vi "VarArray_Find elements.vi"(8 "Error In":errorcluster, 9 "Select Array In":variant[](array[variant]), 11 "Array In":variant[](array[variant])) -> (0 "Error Out":errorcluster, 1 "Selected Array Out":variant[](array[variant]), 2 "Index Array Out":i32[](array[numeric]), 3 "Array Out":variant[](array[variant]))   [LabVIEW 2015]
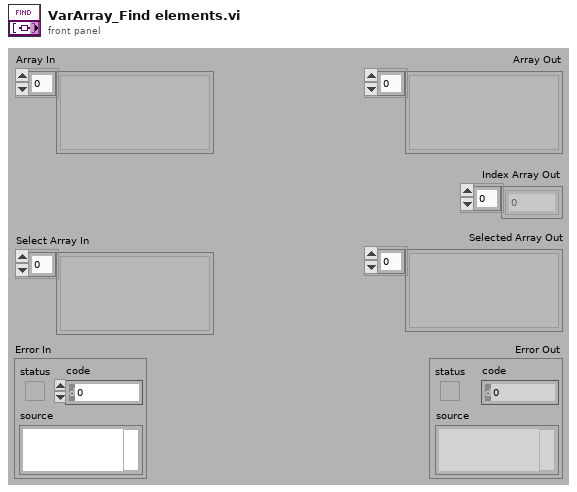
[diagram p1: front panel]
types:
  T1 = typedef "Type Descriptor Enumeration.ctl" = enum8{"<Null>", "I8", "I16", "I32", "I64", "U8", "U16", "U32", "U64", "SGL", "DBL", "EXT", "CSG", "CDB", "CXT", "0x0F", "0x10", "0x11", "0x12", "0x13", "0x14", "Enum U8", "Enum U16", "Enum U32", "Enum U64", "SGL PQ", "DBL PQ", "EXT PQ", "CSG PQ", "CDB PQ", "CXT PQ", "0x1F", "0x20", "Boolean", "0x22", "0x23", "0x24", "0x25", "0x26", "0x27", "0x28", "0x29", "0x2A", "0x2B", "0x2C", "0x2D", "0x2E", "0x2F", "String", "0x31", "Path", "Pict", "0x34", "0x35", "0x36", "DAQ", "0x38", "0x39", "0x3A", "0x3B", "0x3C", "0x3D", "0x3E", "0x3F", "Array", "0x41", "0x42", "0x43", "0x44", "0x45", "0x46", "0x47", "0x48", "0x49", "0x4A", "0x4B", "0x4C", "0x4D", "0x4E", "0x4F", "Cluster", "0x51", "0x52", "Variant", "Waveform", "0x55", "0x56", "0x57", "0x58", "0x59", "0x5A", "0x5B", "0x5C", "0x5D", "0x5E", "0x5F", "0x60", "0x61", "0x62", "0x63", "0x64", "0x65", "0x66", "0x67", "0x68", "0x69", "0x6A", "0x6B", "0x6C", "0x6D", "0x6E", "0x6F", "Refnum"}
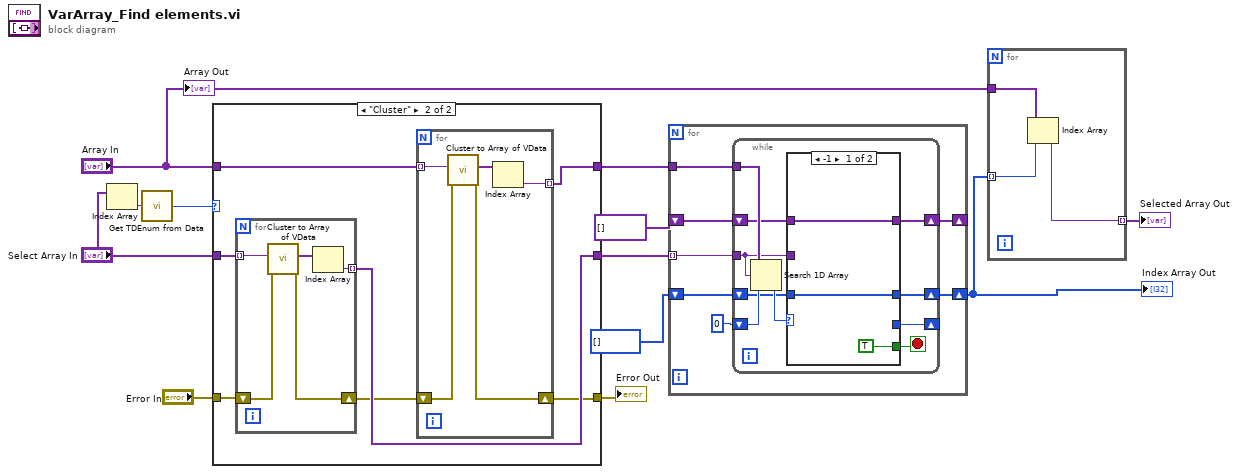
[diagram p0: block diagram]
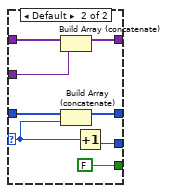
[diagram p3: hidden frame]
diagram:
  n1 = Index Array(array="Select Array In") -> (element=w12:variant)  [unwired: 1 in]
  n2 = call "Get TDEnum from Data.vi"("Data"=w12) -> ("Type Descriptor Enumeration"=w8:T1)  [unwired: 4 in]
  n3 = case shown="\"Cluster\"" w8 {
    tunnel: [w14 w19] -> w11
    tunnel: "Select Array In" -> [w14 w21]
    tunnel: [w15 w20] -> w9
    tunnel: "Array In" -> [w15 w22]
    tunnel: "Error In" -> [w13 w18]
    tunnel: [w13 w16] -> w1
    frame Default {
    }
    frame "Cluster" {
      n4 = for {
        tunnel: w21 -> [w27] mode=indexing
        tunnel: [w25] -> w19 mode=indexing
        shift-right: [w23] -> w17
        shift-left: w18 -> [w24]
        n5 = call "Cluster to Array of VData.vi"("error in (no error)"=w24, "Cluster"=w27) -> ("error out"=w23:errorcluster, "Array of VData"=w26:variant[])  [unwired: 8 in]
        n6 = Index Array(array=w26) -> (element=w25:variant)  [unwired: 1 in]
      }
      n7 = for {
        tunnel: w22 -> [w32] mode=indexing
        tunnel: [w30] -> w20 mode=indexing
        shift-right: [w28] -> w16
        shift-left: w17 -> [w29]
        n8 = call "Cluster to Array of VData.vi"("error in (no error)"=w29, "Cluster"=w32) -> ("error out"=w28:errorcluster, "Array of VData"=w31:variant[])  [unwired: 8 in]
        n9 = Index Array(array=w31) -> (element=w30:variant)  [unwired: 1 in]
      }
    }
  }
  "Error Out" <- w1
  n10 = for {
    tunnel: w11 -> [w39] mode=indexing
    tunnel: w9 -> [w38]
    shift-right: [w36] -> w4
    shift-left: i32[] [] -> [w35]
    shift-right: [w34] -> _
    shift-left: variant[] [] -> [w33]
    n11 = while {
      tunnel: w39 -> [w42]
      tunnel: w38 -> [w49]
      shift-right: [w48] -> _
      shift-left: 0 -> [w47]
      shift-right: [w45] -> w36
      shift-left: w35 -> [w44]
      shift-right: [w41] -> w34
      shift-left: w33 -> [w40]
      stop <- w43 stop-if-true
      n12 = Search 1D Array(1D array=w49, element=w42, start index (0)=w47) -> (index of element=w46:i32)
      n13 = case shown="-1" w46 {
        selector: w46 -> [_ w57]
        tunnel: [w52 w60] -> w45
        tunnel: [_ w59] -> w48
        tunnel: w44 -> [w52 w58]
        tunnel: [TRUE FALSE] -> w43
        tunnel: w42 -> [_ w55]
        tunnel: [w50 w54] -> w41
        tunnel: w40 -> [w50 w53]
        frame -1 {
        }
        frame Default {
          n14 = Build Array (concatenate)(w53, w55) -> (w54:variant[])
          n15 = Build Array (concatenate)(w58, w57) -> (w60:i32[])
          n16 = Increment(x=w57) -> (x+1=w59:i32)
        }
      }
    }
  }
  "Index Array Out" <- w4
  n17 = for {
    tunnel: "Array In" -> [w63]
    tunnel: w4 -> [w62] mode=indexing
    tunnel: [w61] -> w3 mode=indexing
    n18 = Index Array(array=w63, index=w62) -> (element=w61:variant)
  }
  "Selected Array Out" <- w3
  "Array Out" <- "Array In"
